vi "Cleanup.vi"(8 "error in (no error)":errorcluster, 10 "System In":refnum<class "bt_System.lvclass">, 11 "Node in":refnum<class "bt_Composite.lvclass">) -> (0 "error out":errorcluster, 2 "System Out":refnum<class "bt_System.lvclass">, 3 "Node out":refnum<class "bt_Composite.lvclass">)   [LabVIEW 2021, in "BT.lvlib" / "bt_Composite.lvclass"]
uses:
  bt_Composite.lvclass
  abs_System/bt_System.lvclass
  bt_Composite.lvclass/bt_Composite.ctl
  abs_Node/bt_Node.lvclass
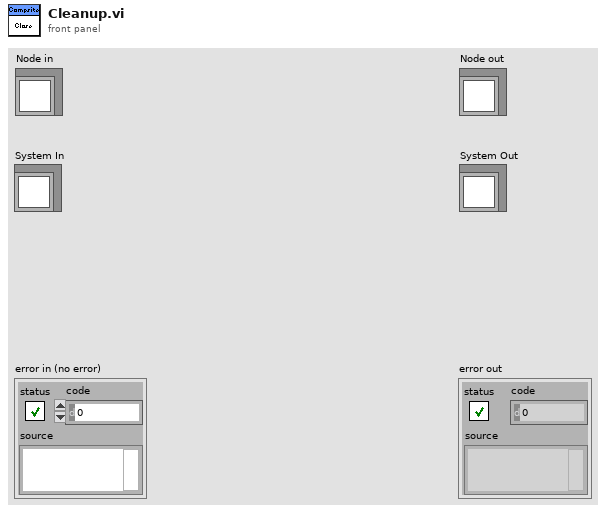
[diagram p1: front panel]
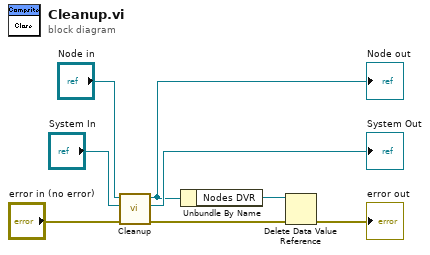
[diagram p0: block diagram]
diagram:
  n1 = call-parent "Cleanup.vi"("error in (no error)"="error in (no error)", "System In"="System In", "Node in"="Node in") -> ("error out"=w3:errorcluster, "System Out"=→"System Out":refnum<class "bt_System.lvclass">, "Node out"=w4:refnum<class "bt_Composite.lvclass">)  [unwired: 6 in]
  "Node out" <- w4
  n2 = Unbundle By Name(w4) -> ("Nodes DVR"=w2:refnum<data-value>)
  n3 = Delete Data Value Reference(data value reference=w2, error in=w3) -> (error out=→"error out":errorcluster)  [unwired: 1 out]
